vi "Get Directory Size On Disk.vi"(8 "error in":errorcluster, 11 "Path":path) -> (0 "error out":errorcluster, 2 "Bytes":i32, 3 "dup Path":path)   [LabVIEW 2017, in "G3_Build Process File Utilities.lvlib"]
doc: "Returns the size of this directory including all sub directories. This function is the equivalent of righ clicking on a directory and selecting properties."
uses:
  G3_Build Process File Utilities.lvlib
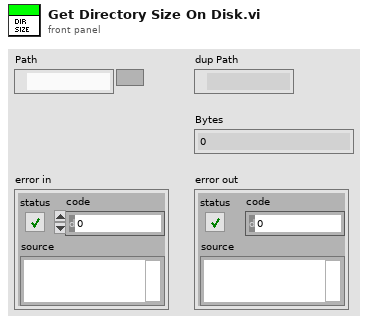
[diagram p1: front panel]
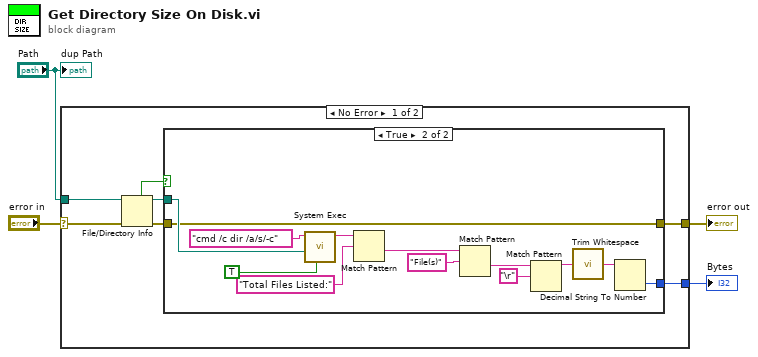
[diagram p0: block diagram]
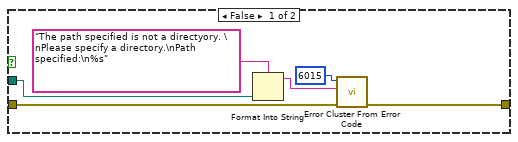
[diagram p2: hidden frame]
diagram:
  n1 = case shown="No Error" "error in" {
    selector: "error in" -> [w7 w31]
    tunnel: "Path" -> [w11 _]
    tunnel: [w8 _] -> w3
    tunnel: [w5 w31] -> w1
    frame No Error {
      n2 = File/Directory Info(path=w11, error in=w7) -> (path out=w9:path, directory=w10:bool, error out=w6:errorcluster)  [unwired: 4 out]
      n3 = case shown="True" w10 {
        tunnel: w9 -> [w14 w30]
        tunnel: [_ w20] -> w8
        tunnel: w6 -> [w17 w19]
        tunnel: [w16 w19] -> w5
        frame False {
          n4 = Format Into String(format string="The path specified is not a directyory. \nPlease specify a directory.\nPath specified:\n%s", w14) -> (resulting string=w13:string)  [unwired: 2 in, 1 out]
          n5 = call <vilib>:"Error Cluster From Error Code.vi"("error in (no error)"=w17, "error message (\"\")"=w13, "error code (0)"=6015) -> ("error out"=w16:errorcluster)  [unwired: 6 in]
        }
        frame True {
          n6 = call <vilib>:"System Exec.vi"("run minimized? (F)"=TRUE, "working directory"=w30, "command line"="cmd /c dir /a/s/-c") -> ("standard output"=w28:string)  [unwired: 5 in, 3 out]
          n7 = Match Pattern(string=w28, regular expression="Total Files Listed:") -> (after substring=w26:string)  [unwired: 1 in, 3 out]
          n8 = Match Pattern(string=w26, regular expression="File(s)") -> (after substring=w24:string)  [unwired: 1 in, 3 out]
          n9 = Match Pattern(string=w24, regular expression="\r") -> (before substring=w22:string)  [unwired: 1 in, 3 out]
          n10 = call <vilib>:"Trim Whitespace.vi"("string"=w22) -> ("trimmed string"=w21:string)  [unwired: 1 in]
          n11 = Decimal String To Number(string=w21) -> (number=w20:i32)  [unwired: 2 in, 1 out]
        }
      }
    }
    frame Error {
    }
  }
  "Bytes" <- w3
  "error out" <- w1
  "dup Path" <- "Path"
